vi "repPrepareGoalKickEnemyPlayVSS.vi"(0 "PrepareGoalKickEnemyPlayVSS in":refnum<class "PrepareGoalKickEnemyPlayVSS.lvclass">, 1 "RobotPlacement":T1(array[cluster]), 2 "Game in 2":refnum<class "Game.lvclass">, 3 "error in (no error)":errorcluster) -> (7 "PrepareGoalKickEnemyPlayVSS out":refnum<class "PrepareGoalKickEnemyPlayVSS.lvclass">, 8 "RobotPlacement 2":T1(array[cluster]), 10 "error out":errorcluster)   [LabVIEW 2023, in "PrepareGoalKickEnemyPlayVSS.lvclass"]
uses:
  PrepareGoalKickEnemyPlayVSS.lvclass
  Game_class/Game.lvclass
  Game_class/Game.lvclass/Game.ctl
  Object_class/Object.lvclass/Object.ctl
  Game_class/Read FieldRef.vi
  Game_class/Read BallRef.vi
  Game_class/Read EnemyRef.vi
  Team_class/Read RobotRef.vi
  Object_class/Read y.vi
  Ball_class/Ball.lvclass
  Field_class/Field.lvclass
  Enemy_class/Enemy.lvclass
  Robot_class/Robot.lvclass
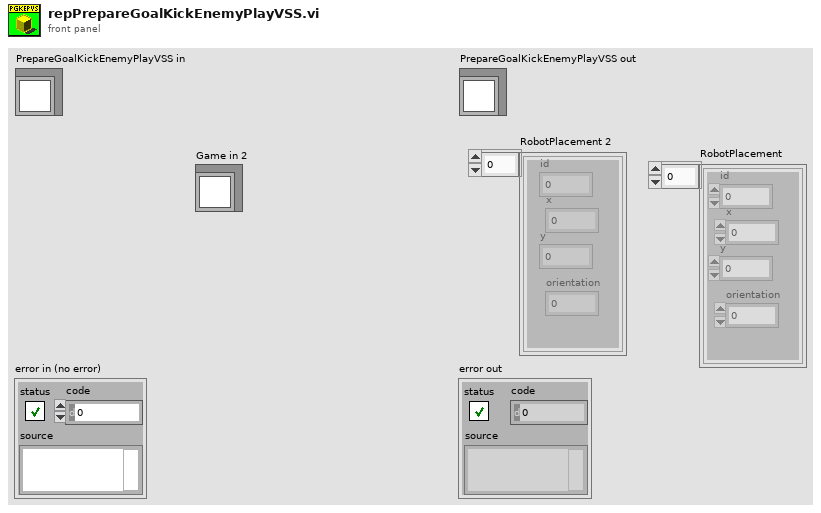
[diagram p1: front panel]
types:
  T1 = cluster{"id":i32, "x":dbl, "y":dbl, "orientation":dbl}[]
  T2 = cluster{"id":i32, "x":dbl, "y":dbl, "orientation":dbl}
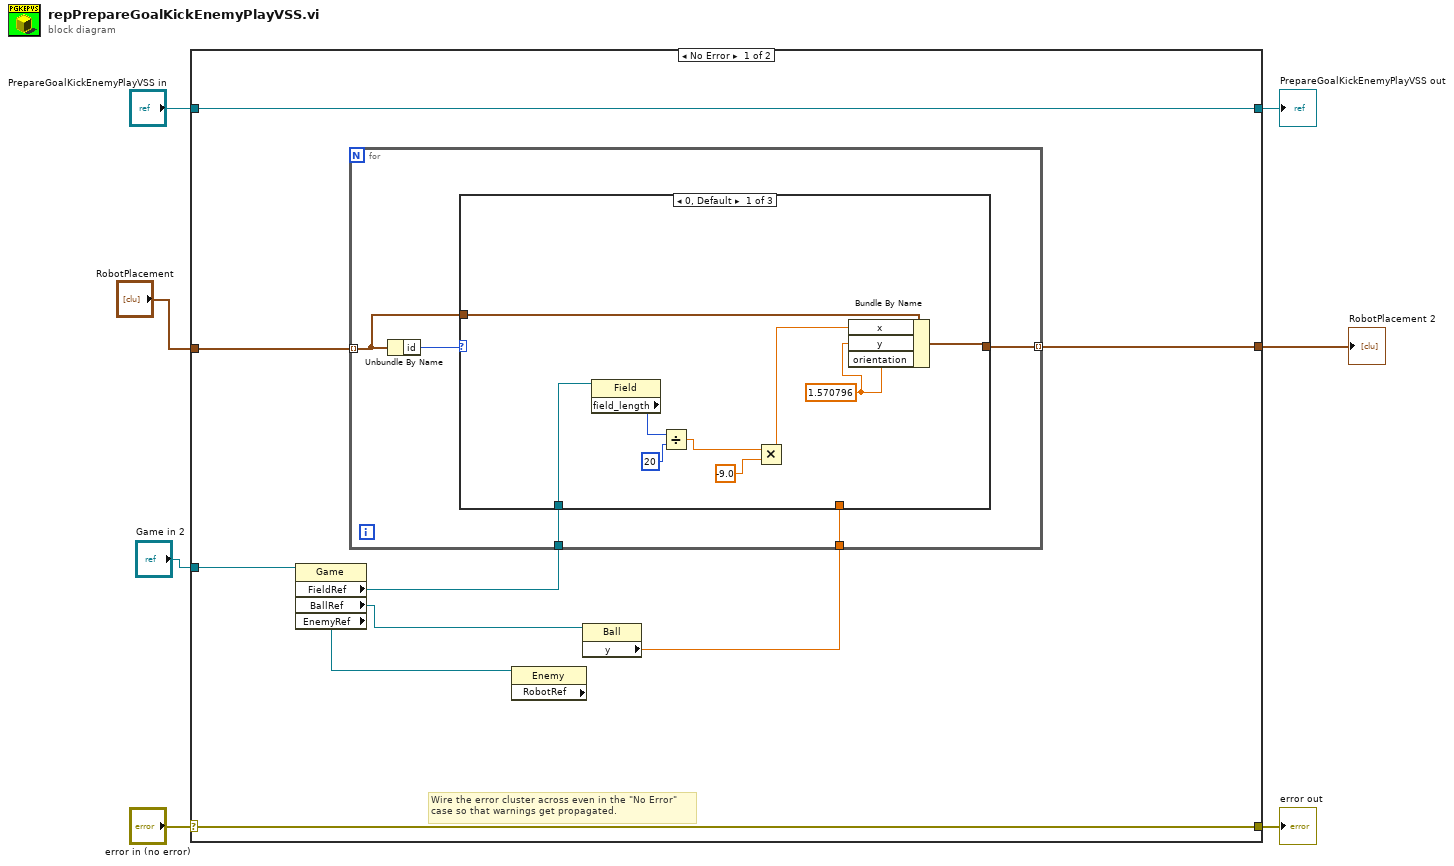
[diagram p0: block diagram]
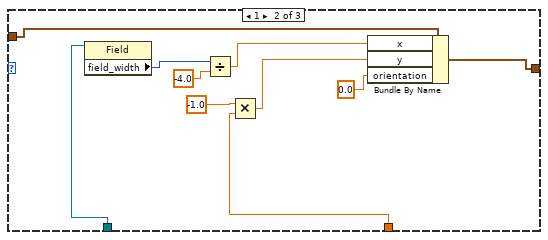
[diagram p2: hidden frame]
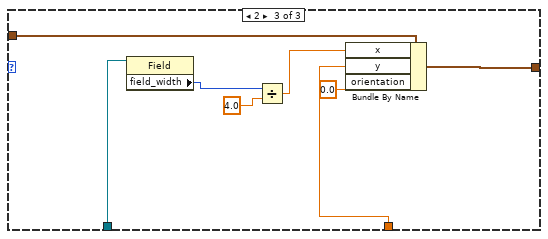
[diagram p3: hidden frame]
diagram:
  n1 = case shown="No Error" "error in (no error)" {
    selector: "error in (no error)" -> [w15 w50]
    tunnel: [w15 w50] -> w6
    tunnel: [w16 w49] -> w4
    tunnel: "PrepareGoalKickEnemyPlayVSS in" -> [w16 w49]
    tunnel: [w13 _] -> w3
    tunnel: "Game in 2" -> [w12 _]
    tunnel: "RobotPlacement" -> [w11 _]
    frame No Error {
      # "Wire the error cluster across even in the \"No Error\"\ncase so that warnings get propagated."
      n2 = property class="Game"(reference=w12) -> ("FieldRef"=w14:refnum<class "Field.lvclass">, "BallRef"=w10:refnum<class "Ball.lvclass">, "EnemyRef"=w8:refnum<class "Enemy.lvclass">)  [unwired: 1 in, 2 out]
      n3 = property class="Enemy" props=["RobotRef"](reference=w8) -> ()  [unwired: 1 in, 3 out]
      n4 = property class="Ball"(reference=w10) -> ("y"=w9:dbl)  [unwired: 1 in, 2 out]
      n5 = for {
        tunnel: [w21] -> w13 mode=indexing
        tunnel: w14 -> [w20]
        tunnel: w11 -> [w18] mode=indexing
        tunnel: w9 -> [w17]
        n6 = Unbundle By Name(w18) -> ("id"=w19:i32)
        n7 = case shown="0, Default" w19 {
          tunnel: [w24 w39 w48] -> w21
          tunnel: w20 -> [w30 w34 w44]
          tunnel: w18 -> [w23 w38 w46]
          tunnel: w17 -> [_ w37 w45]
          frame 0, Default {
            w22 = 1.570796 ("orientation")
            n8 = property class="Field"(reference=w30) -> ("field_length"=w29:i32)  [unwired: 1 in, 2 out]
            n9 = Divide(x=w29, y=20) -> (x/y=w27:dbl)
            n10 = Multiply(x=w27, y=-9.0) -> (x*y=w26:dbl)
            n11 = Bundle By Name(cluster=w23, "x"=w26, "y"=w22, "orientation"=w22) -> (w24:T2)
          }
          frame 1 {
            n12 = property class="Field"(reference=w34) -> ("field_width"=w33:i32)  [unwired: 1 in, 2 out]
            n13 = Divide(x=w33, y=-4.0) -> (x/y=w31:dbl)
            n14 = Multiply(x=-1.0, y=w37) -> (x*y=w35:dbl)
            n15 = Bundle By Name(cluster=w38, "x"=w31, "y"=w35, "orientation"=0.0 ("x")) -> (w39:T2)
          }
          frame 2 {
            n16 = property class="Field"(reference=w44) -> ("field_width"=w42:i32)  [unwired: 1 in, 2 out]
            n17 = Divide(x=w42, y=4.0) -> (x/y=w41:dbl)
            n18 = Bundle By Name(cluster=w46, "x"=w41, "y"=w45, "orientation"=0.0) -> (w48:T2)
          }
        }
      }
    }
    frame Error {
    }
  }
  "error out" <- w6
  "PrepareGoalKickEnemyPlayVSS out" <- w4
  "RobotPlacement 2" <- w3
